vi "Button Logic.vi"(4 "Set Mode":enum16{"Noop", "Button", "Switch"}(ring), 7 "In":bool, 9 "Button In":T1) -> (0 "Trailing":bool, 1 "Leading":bool, 2 "Out":bool, 3 "Button Out":T1)   [LabVIEW 2012, in "femtoRoboLib.lvlib"]
uses:
  femtoRoboLib.lvlib
  Button Control.ctl
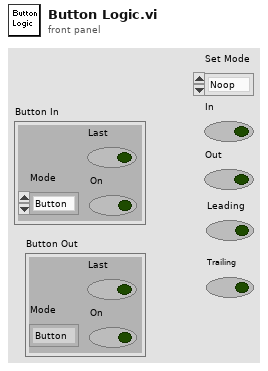
[diagram p1: front panel]
types:
  T1 = typedef "femtoRoboLib.lvlib/Button Control.ctl" = cluster{"Last":bool, "Mode":enum16{"Button", "Switch"}, "On":bool}
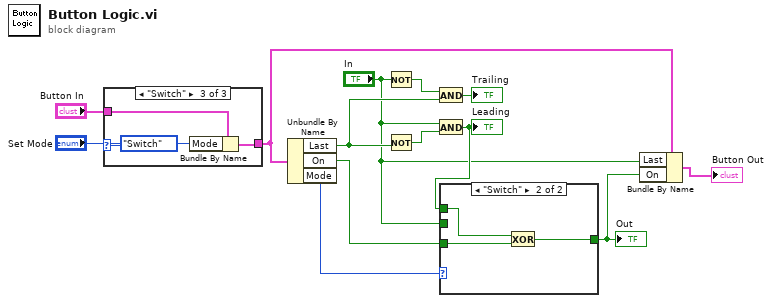
[diagram p0: block diagram]
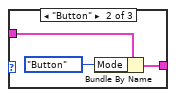
[diagram p3: hidden frame]
diagram:
  n1 = case shown="\"Switch\"" "Set Mode" {
    tunnel: "Button In" -> [w14 w17 w18]
    tunnel: [w14 w16 w19] -> w7
    frame "Noop", Default {
    }
    frame "Button" {
      n2 = Bundle By Name(cluster=w17, "Mode"=enum16{"Button", "Switch"}."Button") -> (w16:T1)
    }
    frame "Switch" {
      n3 = Bundle By Name(cluster=w18, "Mode"=enum16{"Button", "Switch"}."Switch") -> (w19:T1)
    }
  }
  n4 = Unbundle By Name(w7) -> ("Last"=w5:bool, "On"=w4:bool, "Mode"=w10:enum16{"Button", "Switch"})
  n5 = Not(x="In") -> (.not. x?=w13:bool)
  n6 = Not(x=w5) -> (.not. x?=w9:bool)
  n7 = And(x=w13, y=w5) -> (x .and. y?=→"Trailing":bool)
  n8 = And(x="In", y=w9) -> (x .and. y?=w2:bool)
  "Leading" <- w2
  n9 = case shown="\"Switch\"" w10 {
    tunnel: "In" -> [w21 _]
    tunnel: [w21 w22] -> w3
    tunnel: w2 -> [_ w23]
    tunnel: w4 -> [_ w24]
    frame "Button", Default {
    }
    frame "Switch" {
      n10 = Exclusive Or(1:w24, 2:w23) -> (0:w22:bool)
    }
  }
  "Out" <- w3
  n11 = Bundle By Name(cluster=w7, "Last"="In", "On"=w3) -> (→"Button Out":T1)
